vi "Read LS ActorQ.vi"(8 "error in (no error)":errorcluster, 11 "Chassis Tasks in":refnum<class "Chassis Tasks.lvclass">) -> (0 "error out":errorcluster, 2 "Actor Framework.lvlib:Message Enqueuer":refnum<class "Message Enqueuer.lvclass">, 3 "Chassis Tasks out":refnum<class "Chassis Tasks.lvclass">)   [LabVIEW 2018, in "Data Acquisition.lvlib" / "Chassis Tasks.lvclass"]
uses:
  Chassis Tasks.lvclass
  <vilib>/ActorFramework/Message Enqueuer/Message Enqueuer.lvclass
  Chassis Tasks.lvclass/Chassis Tasks.ctl
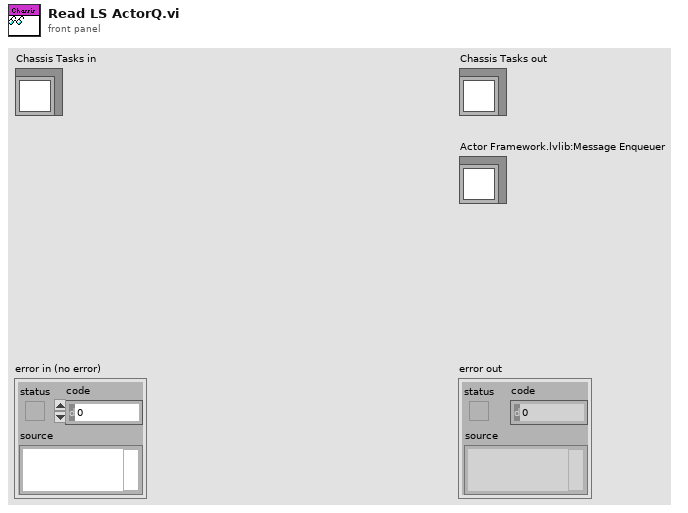
[diagram p1: front panel]
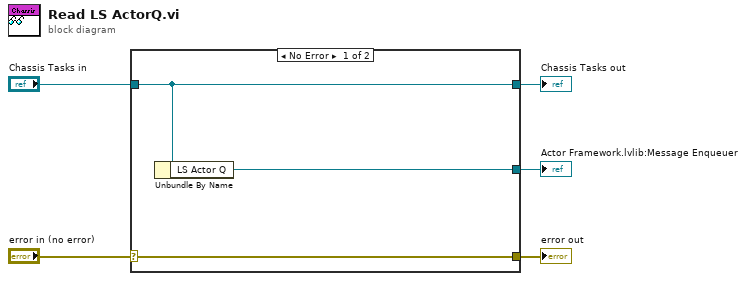
[diagram p0: block diagram]
diagram:
  n1 = case shown="No Error" "error in (no error)" {
    selector: "error in (no error)" -> [w8 w9]
    tunnel: [w8 w9] -> w4
    tunnel: [w7 w10] -> w2
    tunnel: "Chassis Tasks in" -> [w7 w10]
    tunnel: [w6 _] -> w1
    frame No Error {
      n2 = Unbundle By Name(w7) -> ("LS Actor Q"=w6:refnum<class "Message Enqueuer.lvclass">)
    }
    frame Error {
    }
  }
  "error out" <- w4
  "Chassis Tasks out" <- w2
  "Actor Framework.lvlib:Message Enqueuer" <- w1
